vi "AlliGator Create Source Image Contour ROI.vi"(6 "Image Label":string, 7 "ROI Mask":T1, 8 "Error In":errorcluster, 10 "ROI":T2 {"Contours"."Type" items=["No Selection", "Point", "Line", "Rectangle", "Oval", "Polygon", "Freehand Region", "Annulus", "Unused2", "Unused3", "Broken Line", "Freehand Line", "Rotated Rectangle"]}, 11 "Image":T1) -> (0 "Error Out":errorcluster, 2 "Message":string)   [LabVIEW 2021, in "AlliGator ROIs.lvlib"]
doc: "Create new Source Image ROI consisting of the contour of the input ROI."
uses:
  AlliGator ROIs.lvlib
  <vilib>/vision/Image Controls.llb/IMAQ Image.ctl
  AlliGator ROI Manager Actions.ctl
  AlliGator Variables List.ctl
  Image/Named ROI Description.ctl
  <vilib>/Utility/error.llb/Error Cluster From Error Code.vi
  Variant/Variant to Data/Variant to I32.vi
  AlliGator Source Image ROI Storage [SGL] v3.vi
  <vilib>/ErrorRing/Error Ring.xnode
  AlliGator Globals, Variables & Constants.lvlib
  Variant/Variant to Data/Variant to Data.lvlib
  Image/Image.lvlib
panel:
  # "see the AlliGator License on the block diagram (Ctrl+E or Window:Show Block Diagram)"
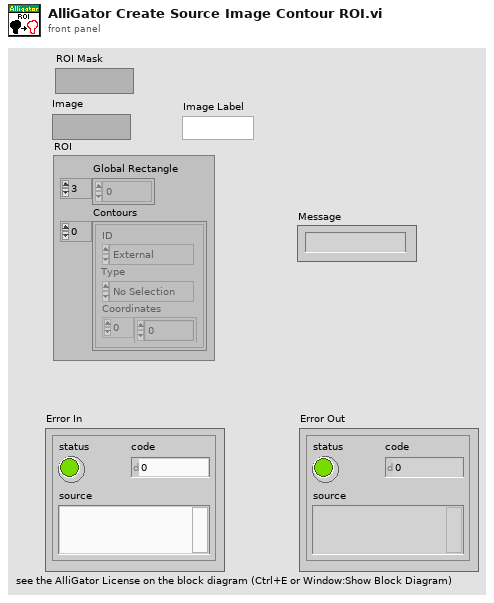
[diagram p1: front panel]
types:
  T1 = typedef "IMAQ Image.ctl" = refnum<image>
  T2 = typedef "ROI Descriptor" = cluster{"Global Rectangle":i32[], "Contours":cluster{"ID":enum32{"External", "Internal"}, "Type":u32, "Coordinates":i32[]}[]}
  T3 = typedef "Image.lvlib/Named ROI Description.ctl" = cluster{"ROI Descriptor":T2, "ROI Name":string, "Overlay Color":u32}
  T4 = typedef "AlliGator Globals, Variables & Constants.lvlib/AlliGator Variables List.ctl" = enum16{"---- GUI ----", "Initialization Status", "State Indicators Refnum", "Original AlliGator Menu Items", "Current Action Loop State", "Script in progress", "Playback", "Loop Playback", "Search ROI Used", "Search ROI", "Decay Graph Max Legend Size", "Intensity Graph Max Legend Size", "Decay Statistics Graph Max Legend Size", "Phasor Graph Max Legend Size", "Phasor Ratio Graph Max Legend Size", "Lifetime Graph Max Legend Size", "---- Files ----", "Export Dataset Frames as Individual Files", "Show Batch Export Help Balloons", "Frames in Dataset", "ptu File Frame Start Indices", "Current Frame in Dataset", "Current Frame Timestamp", "------ Python Plugins ------", "Python Plugins Information", "Python Session", "Valid Python Session?", "---- Source Image ----", "Dataset Loaded", "Dataset Metadata", "Dataset Channel", "Dataset Data Description", "Background Dataset Metadata", "Background Dataset Channel", "Background Dataset Data Description", "Background File Subtraction", "Background File Path", "Background File Pile-up Correction", "Background File Pixel Well Capacity", "Background File Scaling Factor", "Source Image ROIs", "Current Source Image ROI", "Source Image ROI Event Refnum", "X_Source Image Display Range", "X_Source Image Palette Information", "Source Image Palette List", "Source Image Scale", "Current Dataset Load Settings", "Source Image:ROI Overlay Color", "---- Image Profile Window ----", "Image Profile:Overlay ROI in Source Image", "Image Profile Window Event Refnum", "Image Profile:IntensityType", "Image Profile:Intensity Average Type", "Image Profile:Intensity-weighted SDV", "Image Profile:Box Profile Type", "Image Profile Window Open", "Image Profile:Plotted Fit Parameter", "X_Type of Displayed Image", "X_Time Gate Slider", "Dataset Path", "Source Image Overlay to Erase", "Is Displayed Image Accumulated", "White Light Image Modified", "Mask Image Modified", "Macrotime Gate Separation", "------ Phasor Graph -------", "Phasor Graph:Show Line", "---- Phasor Plot ---", "Phasor Plot Parameters Changed", "FLI Dataset Modified since last Phasor Plot Calculation", "Phasor Harmonics Data", "Selected Phasor Harmonics", "Phasor Harmonic Manager Event Refnum", "Phasor Plot ROIs", "Current Phasor Plot ROI", "Phasor Plot ROI Event Refnum", "Phasor Plot Image Reference Points", "Phasor Plot Computed", "Phasor Plot Palette Information", "Phasor Plot Palette List", "Phasor Ratio Palette Information", "Phasor Ratio Palette List", "Phasor Image Scale", "Phasor Plot Image Overlay to Erase", "Phasor Plot Image Elements to Update", "Current Phasor Plot Calculation Parameters", "Current Phasor Calibration Options", "Reset Cumulated Phasor Plot", "Phasor Ratio Reference 1", "Phasor Ratio Lifetime Reference 1", "Phasor Ratio Reference 1 Frequency", "Phasor Ratio Reference 2", "Phasor Ratio Lifetime Reference 2", "Phasor Ratio Reference 2 Frequency", "---- Decay Analysis ----", "Number of Selected Decays to Fit", "LS Fit Results", "LAR Fit Results", "BS Fit Results", "Last Decay Max - Min", "Best Fit Parameters", "Best Fit Parameter Names", "Actual Size X", "Actual Size Y", "Binning X", "Binning Y", "Actual # Gates", "Dataset Number", "Gates to...", "Gates Skipped", "Gates to keep", "Gate Step", "Gate Separation", "Reversed Gates", "Pile-up Correction", "Pixel Well Capacity", "Background Subtracted", "Background Subtraction Method", "Background Definition Range", "Background File (deprecated)", "Number of Dataset Accumulated", "Array of Accumulated Dataset Paths", "Do Averaged Datasets", "Destination File Path", "Process Plot Target", "Use 1/D as Phasor Frequency", "---- Decay Fit Parameter Map -----", "Decay Fit Parameter Map Palette Information", "Decay Fit Parameter Map Palette List", "Local Decay Graph Window Event Refnum", "------- Local Decay Window ---------", "Use normalized IRF for convolution", "----- Miscellaneous ----", "Skippable Dialog Windows Status"}
  T5 = typedef "AlliGator ROIs.lvlib/AlliGator ROI Manager Actions.ctl" = enum16{"Undefined", "Delete Current ROI", "Delete All Unselected ROIs", "Delete Multiple ROIs", "Delete All ROIs", "Swap ROIs", "Insert ROI", "Update Current ROI Descriptor", "Rename Current ROI", "Store New ROI", "Store Multiple ROIs", "Select Next ROI", "Select Previous ROI", "Find Selected ROI", "Show All ROIs", "Update ROI Manager Window", "Merge All ROIs", "Unmerge ROI", "Set Selected ROI by ID"}
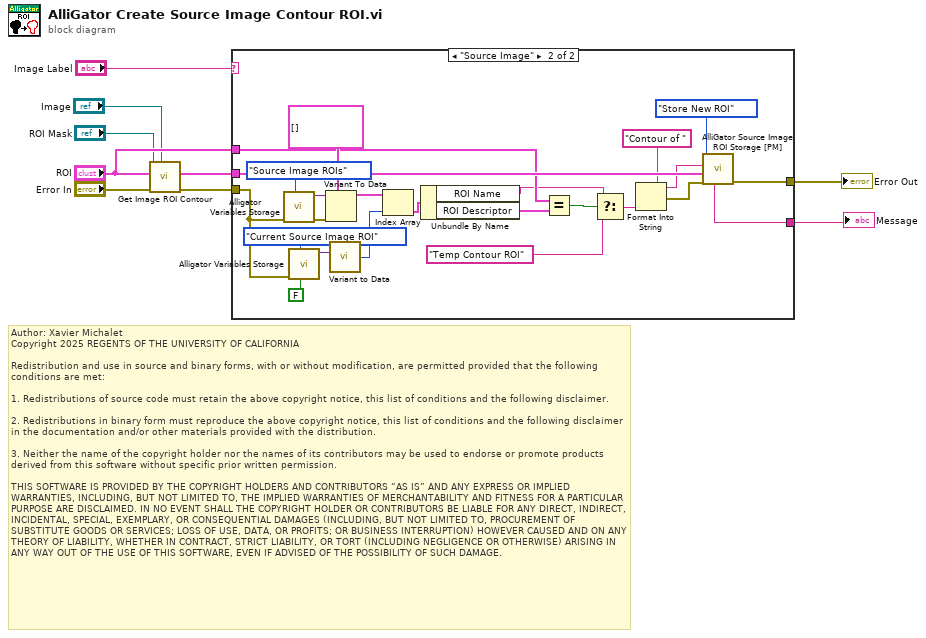
[diagram p0: block diagram]
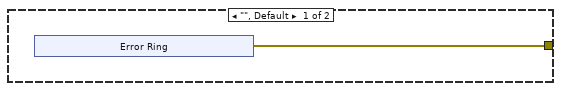
[diagram p2: hidden frame]
diagram:
  # "Author: Xavier Michalet\nCopyright 2025 REGENTS OF THE UNIVERSITY OF CALIFORNIA\n\nRedistribution and use in source and binary forms, with or without modification, are permitted provided that the following conditions are met:\n\n1. Redistributions of source code must retain the above copyright notice, this list of conditions and the following disclaimer.\n\n2. Redistributions in binary form must reproduce the above copyright notice, this list of conditions and the following disclaimer in the documentation and/or other materials provided with the distribution.\n\n3. Neither the name of the copyright holder nor the names of its contributors may be used to endorse or promote products derived from this software without specific prior written permission.\n\nTHIS SOFTWARE IS PROVIDED BY THE COPYRIGHT HOLDERS AND CONTRIBUTORS “AS IS” AND ANY EXPRESS OR IMPLIED WARRANTIES, INCLUDING, BUT NOT LIMITED TO, THE IMPLIED WARRANTIES OF MERCHANTABILITY AND FITNESS FOR A PARTICULAR PURPOSE ARE DISCLAIMED. IN NO EVENT SHALL THE COPYRIGHT HOLDER OR CONTRIBUTORS BE LIABLE FOR ANY DIRECT, INDIRECT, INCIDENTAL, SPECIAL, EXEMPLARY, OR CONSEQUENTIAL DAMAGES (INCLUDING, BUT NOT LIMITED TO, PROCUREMENT OF SUBSTITUTE GOODS OR SERVICES; LOSS OF USE, DATA, OR PROFITS; OR BUSINESS INTERRUPTION) HOWEVER CAUSED AND ON ANY THEORY OF LIABILITY, WHETHER IN CONTRACT, STRICT LIABILITY, OR TORT (INCLUDING NEGLIGENCE OR OTHERWISE) ARISING IN ANY WAY OUT OF THE USE OF THIS SOFTWARE, EVEN IF ADVISED OF THE POSSIBILITY OF SUCH DAMAGE."
  n1 = call "Get Image ROI Contour.vi"("Image Model"="Image", "Error In"="Error In", "ROI Descriptor"="ROI", "ROI Mask"="ROI Mask") -> ("Error Out"=w5:errorcluster, "ROI Contour Descriptor"=w4:T2)  [unwired: 6 in]
  n2 = case shown="\"Source Image\"" "Image Label" {
    tunnel: [w10 w38] -> w8
    tunnel: w4 -> [_ w37]
    tunnel: w5 -> [_ w28]
    tunnel: "ROI" -> [_ w19]
    tunnel: [_ w29] -> w7
    frame "", Default {
      n3 = xnode "Error Ring"() -> ("error out"=w10:errorcluster)
    }
    frame "Source Image" {
      n4 = call "Alligator Variables Storage.vi"("AlliGator Variable"=AlliGator_Variables_List."Source Image ROIs" ("Alligator Variable"), "Error In"=w28) -> ("Error Out"=w25:errorcluster, "Data out"=w26:variant)  [unwired: 7 in, 1 out]
      n5 = call "Alligator Variables Storage.vi"("Get(F)/Set"=FALSE, "AlliGator Variable"=AlliGator_Variables_List."Current Source Image ROI" ("Alligator Variable"), "Error In"=w28) -> ("Data out"=w35:variant)  [unwired: 6 in, 2 out]
      n6 = Variant To Data(error in=w25, type=T3[] [] ("ROIs"), Variant=w26) -> (data=w23:T3[])  [unwired: 1 out]
      n7 = call-poly "Variant to Data.vi"("Variant"=w35) -> ("Value"=w22:i32)  [unwired: 8 in]
      n8 = Index Array(array=w23, index=w22) -> (element=w21:T3)
      n9 = Unbundle By Name(w21) -> ("ROI Name"=w17:string, "ROI Descriptor"=w20:T2)
      n10 = Equal?(x=w19, y=w20) -> (x = y?=w18:bool)
      n11 = Select(t=w17, s=w18, f="Temp Contour ROI") -> (s? t:f=w16:string)
      n12 = Format Into String(initial string="Contour of ", w16) -> (resulting string=w30:string, error out=w31:errorcluster)  [unwired: 2 in]
      n13 = call-poly "AlliGator Source Image ROI Storage [PM].vi"("Error In"=w31, "Current ROI Descriptor"=w37, "Default Name (\"ROI\")"=w30, "Action"=AlliGator_ROI_Manager_Actions."Store New ROI") -> ("Error Out"=w38:errorcluster, "Message"=w29:string)  [unwired: 1 in, 5 out]
    }
  }
  "Error Out" <- w8
  "Message" <- w7
